vi "Twos Complement Conversion.vi"(7 "Input Method (0:String)":u16(ring) items=["String", "Number"], 9 "Input Number":i32, 10 "Input String":string) -> (2 "Output String":string)   [LabVIEW 2015, in "SDG X Series.lvlib"]
doc: "Converts a negative signed number in a string or as a number and take its two's complement as a 14-bit representation, then convert it back to hexadecimal in a string, arranged in little endian order."
uses:
  <instrlib>/SDG X Series/SDG X Series.lvlib
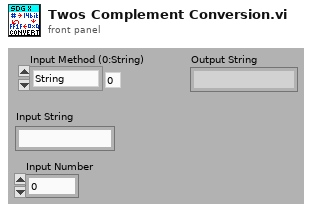
[diagram p1: front panel]
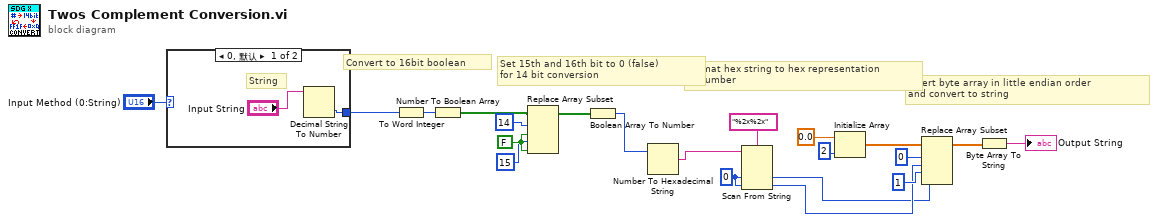
[diagram p0: block diagram]
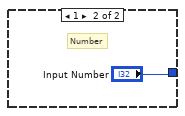
[diagram p2: hidden frame]
diagram:
  w13 = 0 ("default value 1")
  w20 = FALSE
  # "Insert byte array in little endian order\nand convert to string"
  # "Format hex string to hex representation\nof number"
  # "Set 15th and 16th bit to 0 (false)\nfor 14 bit conversion"
  # "Convert to 16bit boolean"
  n1 = case shown="0, 默认" "Input Method (0:String)" {
    tunnel: [w22 "Input Number"] -> w1
    frame 0, Default {
      # "String"
      n2 = Decimal String To Number(string="Input String") -> (number=w22:i32)  [unwired: 2 in, 1 out]
    }
    frame 1 {
      # "Number"
    }
  }
  n3 = To Word Integer(number=w1) -> (16bit integer=w21:i16)
  n4 = Number To Boolean Array(number=w21) -> (Boolean array=w17:bool[])
  n5 = Replace Array Subset(array=w17, new element #1=w20, index #1=14, new element #2=w20, index #2=15) -> (w16:bool[])
  n6 = Boolean Array To Number(Boolean array=w16) -> (number=w15:u32)
  n7 = Number To Hexadecimal String(2:w15) -> (0:w3:string)  [unwired: 1 in]
  n8 = Scan From String(format string="%2x%2x", input string=w3, default 1=w13, default 2=w13) -> (output 1=w4:i32, output 2=w5:i32)  [unwired: 2 in, 3 out]
  n9 = Initialize Array(0.0 ("element"), 2) -> (w11:dbl[])
  n10 = Replace Array Subset(array=w11, new element #1=w5, index #1=0, new element #2=w4, index #2=1) -> (w8:dbl[])
  n11 = Byte Array To String(unsigned byte array=w8) -> (string=→"Output String":string)
